vi "myRIO_BRig_Host_parse_dataTrial__read__compare__v2.vi"(7 "input_maxTrials_Ctrl":i32, 8 "input_arrayCtrl":i32[][](array[numeric]), 9 "input_idxCtrl":i32, 10 "input_arraySample":i32[][](array[numeric]), 11 "input_idxSample":i32) -> (2 "output_arraySample":i32[][](array[numeric]), 3 "output_idxSample":i32)   [LabVIEW 2014]
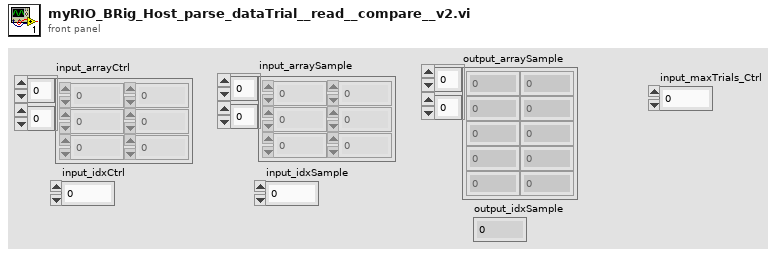
[diagram p1: front panel]
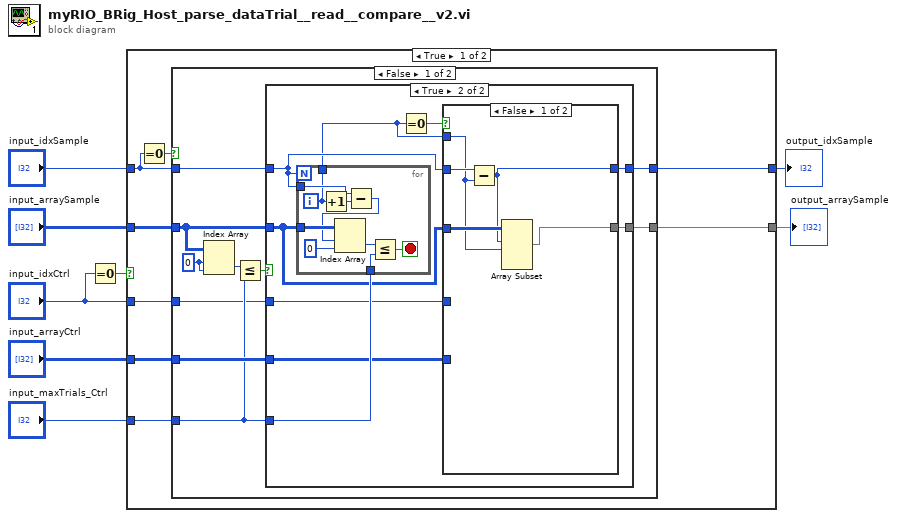
[diagram p0: block diagram]
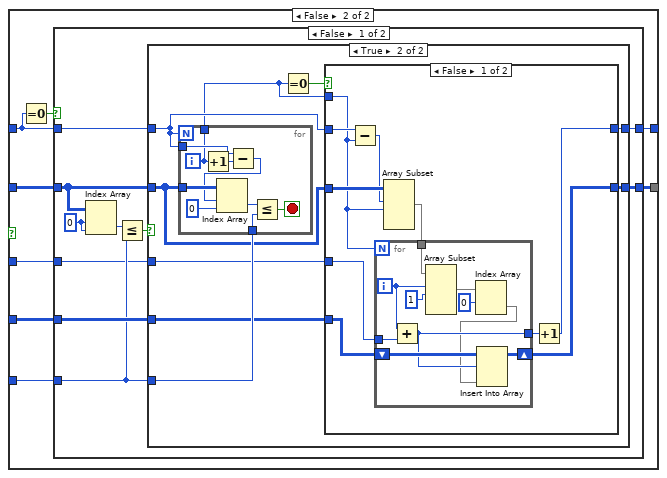
[diagram p5: hidden frame]
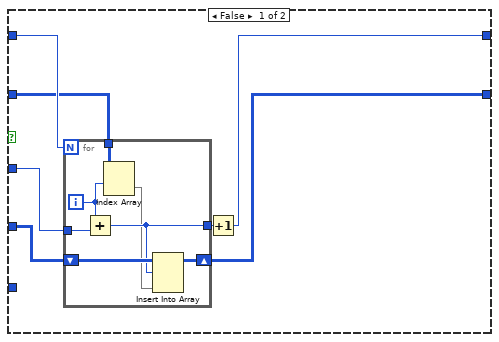
[diagram p6: hidden frame]
diagram:
  n1 = Equal To 0?(x="input_idxCtrl") -> (x = 0?=w8:bool)
  n2 = case shown="True" w8 {
    tunnel: "input_idxSample" -> [w15 w62]
    tunnel: "input_arraySample" -> [w14 w60]
    tunnel: [w9 w61] -> w1
    tunnel: [w13 w59] -> w5
    tunnel: "input_maxTrials_Ctrl" -> [w12 w58]
    tunnel: "input_arrayCtrl" -> [w11 w57]
    tunnel: "input_idxCtrl" -> [w10 w56]
    frame True {
      n3 = Equal To 0?(x=w15) -> (x = 0?=w16:bool)
      n4 = case shown="False" w16 {
        tunnel: w15 -> [w20 w55]
        tunnel: [w21 w55] -> w9
        tunnel: w14 -> [w22 w54]
        tunnel: [w23 w54] -> w13
        tunnel: w12 -> [w18 _]
        tunnel: w11 -> [w19 _]
        tunnel: w10 -> [w17 _]
        frame False {
          w26 = 0 ("index (row)")
          n5 = Index Array(array=w22, index (row)=w26, index (col)=w26) -> (element=w25:i32)
          n6 = Less Or Equal?(x=w25, y=w18) -> (x <= y?=w24:bool)
          n7 = case shown="True" w24 {
            tunnel: [w28 w32] -> w23
            tunnel: w22 -> [w28 w31]
            tunnel: [w27 w33] -> w21
            tunnel: w20 -> [w27 w30]
            tunnel: w19 -> [_ w35]
            tunnel: w18 -> [_ w37]
            tunnel: w17 -> [_ w34]
            frame False {
            }
            frame True {
              n8 = for {
                N: w30 -> [_]
                tunnel: w30 -> [w52]
                tunnel: w31 -> [w51]
                tunnel: w37 -> [w47]
                tunnel: [w45] -> w29
                i -> [w45]
                stop <- w46 stop-if-true
                n9 = Increment(x=w45) -> (x+1=w53:i32)
                n10 = Subtract(x=w52, y=w53) -> (x-y=w50:i32)
                n11 = Index Array(array=w51, index (row)=w50, index (col)=0 ("disabled index (col)")) -> (element=w48:i32)
                n12 = Less Or Equal?(x=w48, y=w47) -> (x <= y?=w46:bool)
              }
              n13 = Equal To 0?(x=w29) -> (x = 0?=w36:bool)
              n14 = case shown="False" w36 {
                tunnel: w35 -> [_ w43]
                tunnel: w34 -> [_ w44]
                tunnel: [w38 w44] -> w33
                tunnel: [w39 w43] -> w32
                tunnel: w31 -> [w41 _]
                tunnel: w30 -> [w42 _]
                tunnel: w29 -> [w40 _]
                frame False {
                  n15 = Subtract(x=w42, y=w40) -> (x-y=w38:i32)
                  n16 = Array Subset(array=w41, index (row)=w38, length (row)=w40) -> (w39:i32[][])  [unwired: 2 in]
                }
                frame True {
                }
              }
            }
          }
        }
        frame True {
        }
      }
    }
    frame False {
      n17 = Equal To 0?(x=w62) -> (x = 0?=w63:bool)
      n18 = case shown="False" w63 {
        tunnel: w62 -> [w68 _]
        tunnel: [w64 w129] -> w61
        tunnel: w60 -> [w69 _]
        tunnel: [w70 w128] -> w59
        tunnel: w58 -> [w66 _]
        tunnel: w57 -> [w67 w128]
        tunnel: w56 -> [w65 w129]
        frame False {
          w73 = 0 ("index (row)")
          n19 = Index Array(array=w69, index (row)=w73, index (col)=w73) -> (element=w72:i32)
          n20 = Less Or Equal?(x=w72, y=w66) -> (x <= y?=w71:bool)
          n21 = case shown="True" w71 {
            tunnel: [w74 w91] -> w70
            tunnel: w69 -> [w77 w90]
            tunnel: [w75 w92] -> w64
            tunnel: w68 -> [w79 w89]
            tunnel: w67 -> [w80 w94]
            tunnel: w66 -> [_ w96]
            tunnel: w65 -> [w78 w93]
            frame False {
              n22 = for {
                N: w79 -> [_]
                shift-right: [w83] -> w74
                shift-left: w80 -> [w84]
                tunnel: w78 -> [w86]
                tunnel: w77 -> [w87]
                tunnel: [w82] -> w76
                i -> [w85]
                n23 = Add(x=w85, y=w86) -> (x+y=w82:i32)
                n24 = Index Array(array=w87, index (row)=w85) -> (element=w81:i32[])  [unwired: 1 in]
                n25 = Insert Into Array(array=w84, index (row)=w82, new element=w81) -> (w83:i32[][])  [unwired: 1 in]
              }
              n26 = Increment(x=w76) -> (x+1=w75:i32)
            }
            frame True {
              n27 = for {
                N: w89 -> [_]
                tunnel: w89 -> [w126]
                tunnel: w90 -> [w125]
                tunnel: w96 -> [w121]
                tunnel: [w119] -> w88
                i -> [w119]
                stop <- w120 stop-if-true
                n28 = Increment(x=w119) -> (x+1=w127:i32)
                n29 = Subtract(x=w126, y=w127) -> (x-y=w124:i32)
                n30 = Index Array(array=w125, index (row)=w124, index (col)=0 ("disabled index (col)")) -> (element=w122:i32)
                n31 = Less Or Equal?(x=w122, y=w121) -> (x <= y?=w120:bool)
              }
              n32 = Equal To 0?(x=w88) -> (x = 0?=w95:bool)
              n33 = case shown="False" w95 {
                tunnel: w94 -> [w100 w117]
                tunnel: w93 -> [w101 w118]
                tunnel: [w98 w118] -> w92
                tunnel: [w97 w117] -> w91
                tunnel: w90 -> [w105 _]
                tunnel: w89 -> [w106 _]
                tunnel: w88 -> [w103 _]
                frame False {
                  n34 = Subtract(x=w106, y=w103) -> (x-y=w104:i32)
                  n35 = Array Subset(array=w105, index (row)=w104, length (row)=w103) -> (w102:i32[][])  [unwired: 2 in]
                  n36 = for {
                    N: w103 -> [_]
                    tunnel: w102 -> [w116]
                    tunnel: w101 -> [w114]
                    shift-right: [w110] -> w97
                    shift-left: w100 -> [w109]
                    tunnel: [w108] -> w99
                    i -> [w113]
                    n37 = Add(x=w113, y=w114) -> (x+y=w108:i32)
                    n38 = Array Subset(array=w116, index (row)=w113, length (row)=1 ("length")) -> (w112:i32[][])  [unwired: 2 in]
                    n39 = Index Array(array=w112, index (row)=0) -> (element=w107:i32[])  [unwired: 1 in]
                    n40 = Insert Into Array(array=w109, index (row)=w108, new element=w107) -> (w110:i32[][])  [unwired: 1 in]
                  }
                  n41 = Increment(x=w99) -> (x+1=w98:i32)
                }
                frame True {
                }
              }
            }
          }
        }
        frame True {
        }
      }
    }
  }
  "output_arraySample" <- w5
  "output_idxSample" <- w1
